vi "Reject Promise.vi"(8 "error in (no error)":errorcluster, 10 "Reason":errorcluster, 11 "Promise in":refnum<class "Promise.lvclass">) -> (0 "error out":errorcluster, 3 "Promise out":refnum<class "Promise.lvclass">)   [LabVIEW 2017, in "Promise Future.lvlib" / "Promise.lvclass"]
uses:
  Promise.lvclass
  E:/Promise/Promise Future/Future/Future.lvclass
  Rejected Future/Rejected Future.lvclass
  Rejected Future/Rejected Future.lvclass/Rejected Future.ctl
  Rejected Future/Write Reason.vi
  Future/Future.lvclass
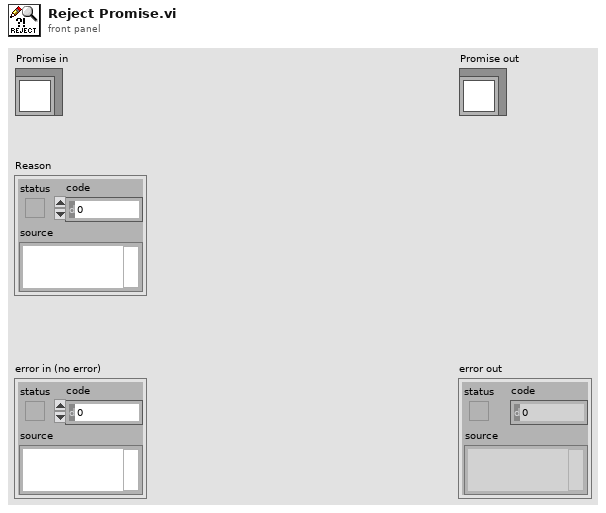
[diagram p1: front panel]
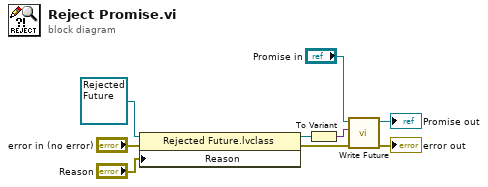
[diagram p0: block diagram]
diagram:
  n1 = property class="Rejected Future.lvclass"(reference=refnum<class "Rejected Future.lvclass"> refnum ("Promise Future.lvlib:Rejected Future.lvclass"), error in="error in (no error)", "Reason"="Reason") -> (reference out=w5:refnum<class "Rejected Future.lvclass">, error out=w4:errorcluster)
  n2 = To Variant(anything=w5) -> (Variant=w3:variant)
  n3 = call "Write Future.vi"("error in (no error)"=w4, "Value"=w3, "Future in"="Promise in") -> ("error out"=→"error out":errorcluster, "Future out"=→"Promise out":refnum<class "Promise.lvclass">)  [unwired: 7 in]
